vi "read_type_descriptor.vi"(5 "type to read":refnum<class "Bytes.lvclass">, 8 "error in (no error)":errorcluster, 9 "length (rest)":i32, 10 "offset (-1)":i32=-1, 11 "LVData in":refnum<class "variant.lvclass">) -> (0 "error out":errorcluster, 2 "Bytes read":refnum<class "Bytes.lvclass">, 3 "LVData out":refnum<class "variant.lvclass">)   [LabVIEW 2020, in "variant.lvlib" / "variant.lvclass"]
uses:
  variant.lvclass
  Bytes/Bytes.lvclass
  variant.lvclass/variant.ctl
  Bytes/Bytes.lvclass/Bytes.ctl
  Bytes/from_byte_array.vi
  Type Descriptor/TD.lvclass
  C:/projects/OpenG-Variant-Data-Library/source/library/Bytes/Bytes.lvclass
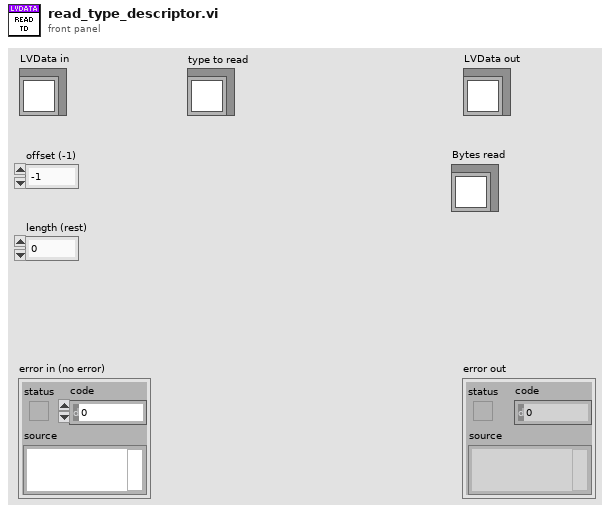
[diagram p1: front panel]
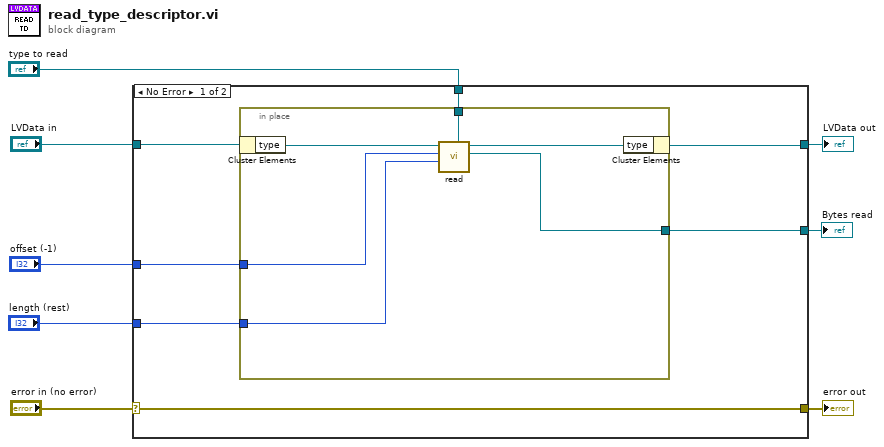
[diagram p0: block diagram]
diagram:
  n1 = case shown="No Error" "error in (no error)" {
    selector: "error in (no error)" -> [w15 w23]
    tunnel: [w15 w23] -> w7
    tunnel: [w13 w22] -> w5
    tunnel: "LVData in" -> [w14 w22]
    tunnel: "offset (-1)" -> [w12 _]
    tunnel: "length (rest)" -> [w11 _]
    tunnel: [w10 _] -> w2
    tunnel: "type to read" -> [w9 _]
    frame No Error {
      n2 = in-place {
        in-place-border: w12 -> [w20]
        in-place-border: w11 -> [w19]
        in-place-border: [w17] -> w10
        in-place-border: w9 -> [w16]
        n3 = in-place-cluster #1(w14) -> ("type"=w21:refnum<class "TD.lvclass">)
        n4 = call "read.vi"("type to read"=w16, "length (-1: rest)"=w19, "offset (-1: current position)"=w20, "Bytes in"=w21) -> ("Bytes read"=w17:refnum<class "Bytes.lvclass">, "Bytes out"=w18:refnum<class "TD.lvclass">)  [unwired: 6 in]
        n5 = in-place-cluster #1("type"=w18) -> (w13:refnum<class "variant.lvclass">)
      }
    }
    frame Error {
    }
  }
  "error out" <- w7
  "LVData out" <- w5
  "Bytes read" <- w2
